vi "Functional Global I32.vi"(9 "Enum":enum16{"Set Data", "Get Data"}(ring), 11 "Integer In":i32) -> (3 "Integer":i32)   [LabVIEW 2014]
panel:
  # "Functional Global Variable (I32)"
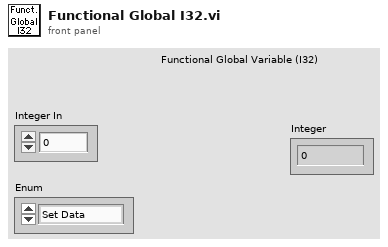
[diagram p1: front panel]
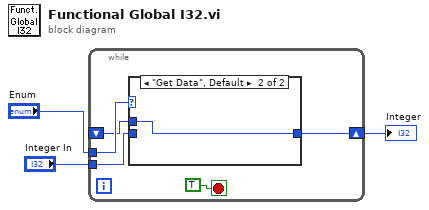
[diagram p0: block diagram]
diagram:
  n1 = while {
    tunnel: "Enum" -> [w8]
    shift-right: [w5] -> w1
    shift-left: _ -> [w4]
    tunnel: "Integer In" -> [w6]
    stop <- TRUE stop-if-true
    n2 = case shown="\"Get Data\", Default" w8 {
      tunnel: w6 -> [w9 _]
      tunnel: [w9 w10] -> w5
      tunnel: w4 -> [_ w10]
      frame "Set Data" {
      }
      frame "Get Data", Default {
      }
    }
  }
  "Integer" <- w1
